vi "ResonanceAnalyzer.vi"() -> ()   [LabVIEW 2014]
uses:
  <vilib>/imath/engines/lvmath2/RunTimeEngine/Managers/WorkSpace/UID Generator.vi
  <vilib>/imathl/engines/lvmath/Functions/Error Handling/Create Error.vi
  <vilib>/imath/engines/lvmath2/RunTimeEngine/LocalVariableDefStatement/MC_LocalVariableDefStatement_Display.vi
  <vilib>/imath/engines/lvmath2/RunTimeEngine/RunTimeType/NIMS_RunTimeType_From StrictType (excl LVString).vi
  <vilib>/imath/engines/lvmath2/RunTimeEngine/BuiltInFunctions/length/NIMS_length(GV).vi
  <vilib>/imath/engines/lvmath2/RunTimeEngine/BuiltInFunctions/ones/NIMS_V=ones(I32,I32).vi
  <vilib>/imath/engines/lvmath2/RunTimeEngine/IndexRead/NIMS V(S).vi
  <vilib>/imath/engines/lvmath2/RunTimeEngine/ErrorHandling/NIMS_Create Error From Enums.vi
  <vilib>/imath/engines/lvmath2/RunTimeEngine/CommandStatement/MC_CommandStatement_break.vi
  <vilib>/imath/engines/lvmath2/RunTimeEngine/Managers/SymbolTable/Clear UID.vi
  <vilib>/imath/engines/lvmath2/RunTimeEngine/Managers/SymbolTable/NIMS_WorkSpace.lvlib
  <vilib>/imath/engines/lvmath2/RunTimeEngine/NodeEndStatement/NIMS_NodeEndStatement_Output.vi
  <vilib>/imath/engines/lvmath2/RunTimeEngine/ErrorHandling/NIMS_Finalize Error.vi
  <vilib>/imath/engines/lvmath2/RunTimeEngine/IndexReplace/NIMS V(S)=S.vi
  <vilib>/Utility/file.llb/Read From Spreadsheet File (DBL).vi
  <vilib>/imath/engines/lvmath2/RunTimeEngine/RangeToken/NIMS_Range_R2 - Integer.vi
  <vilib>/imath/engines/lvmath2/RunTimeEngine/BuiltInFunctions/transpose/NIMS_transpose(GV).vi
  <vilib>/imath/engines/lvmath2/RunTimeEngine/RangeToken/NIMS_Range.vi
  <vilib>/Analysis/NI_AALBase.lvlib
  <vilib>/gmath/NI_Gmath.lvlib
  <vilib>/gmath/NumericalOptimization/Nonlinear Curve Fit LM formula string.vi
panel:
  out "best nonlinear fit":dbl[](array[numeric])
  out "f":dbl[](array[numeric])
  out "A":dbl[](array[numeric])
  out "XY Graph":cluster{"Y":dbl[], "Y":dbl[]}[](graph)
  in  "?":enum32{"Simulation", "Experiment"}(tab)
  in  "Input Parameters":T1
  in  "Filename":path
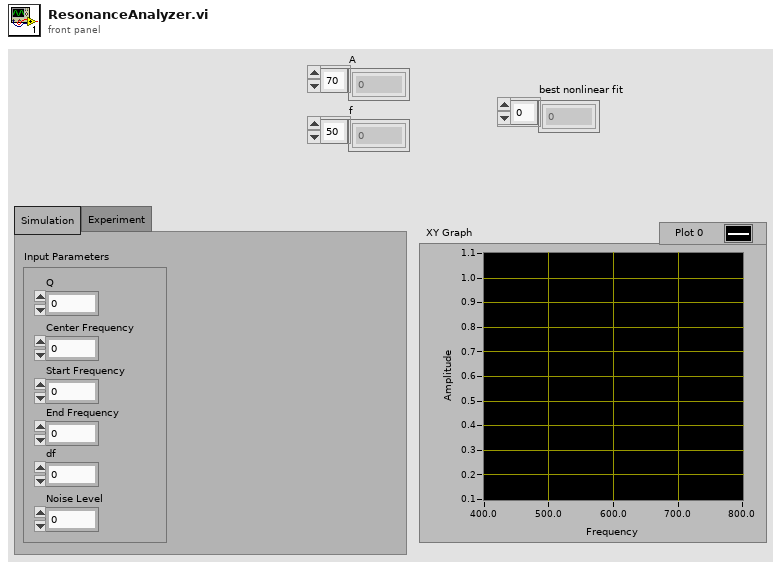
[diagram p1: front panel]
types:
  T1 = cluster{"Q":dbl, "Center Frequency":dbl, "Start Frequency":dbl, "End Frequency":dbl, "df":dbl, "Noise Level":dbl}
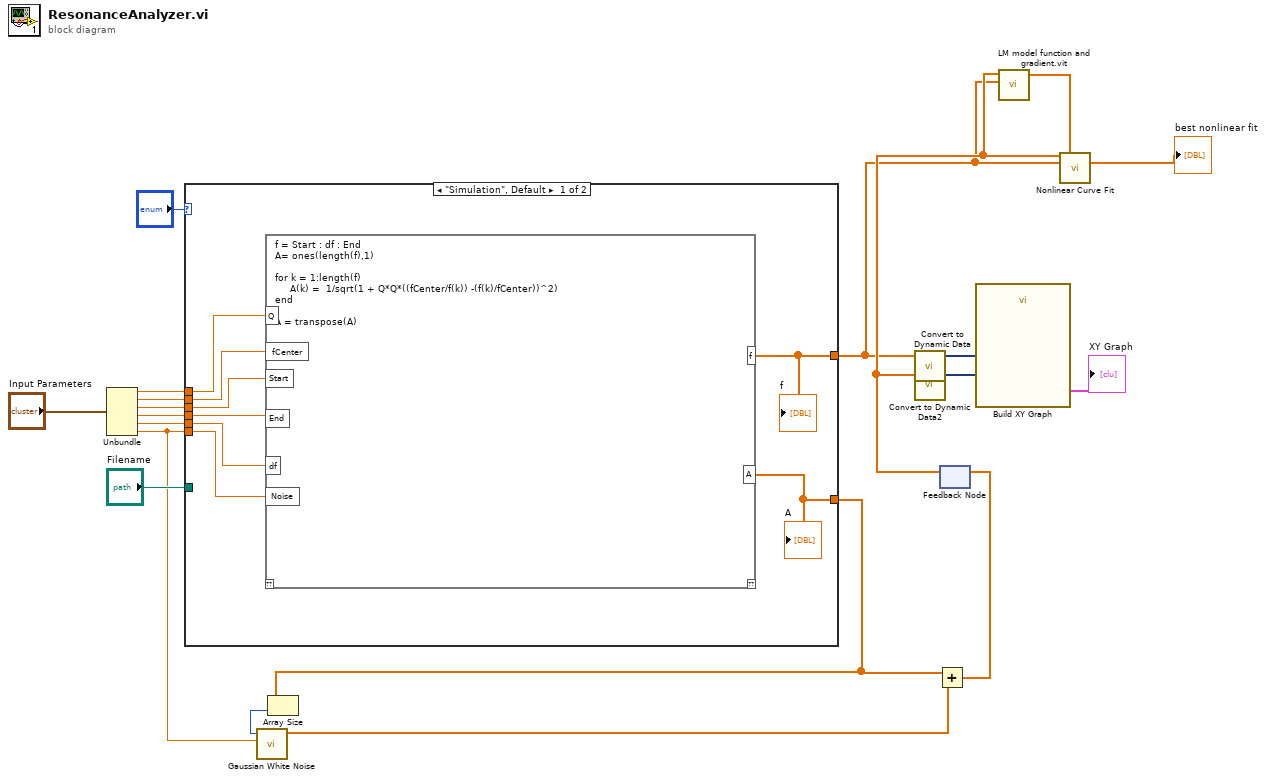
[diagram p0: block diagram]
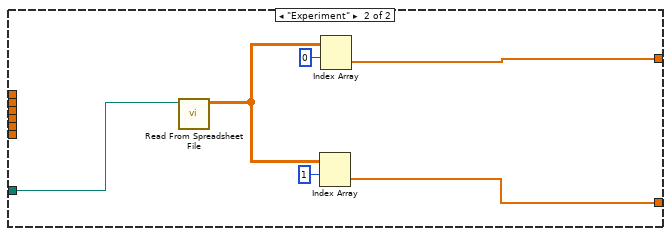
[diagram p2: hidden frame]
diagram:
  n1 = Unbundle("Input Parameters") -> ("Q"=w18:dbl, "Center Frequency"=w17:dbl, "Start Frequency"=w16:dbl, "End Frequency"=w15:dbl, "df"=w14:dbl, "Noise Level"=w9:dbl)
  n2 = case shown="\"Simulation\", Default" "?" {
    tunnel: w18 -> [w28 _]
    tunnel: w17 -> [w27 _]
    tunnel: w16 -> [w26 _]
    tunnel: w15 -> [w25 _]
    tunnel: w14 -> [w24 _]
    tunnel: w9 -> [w23 _]
    tunnel: "Filename" -> [_ w227]
    tunnel: [w21 w223] -> w1
    tunnel: [w22 w222] -> w4
    frame "Simulation", Default {
      n3 = mathscript code="f = Start : df : End\nA= ones(length(f),1)\n\nfor k = 1:length(f)\n     A(k) =  1/sqrt(1 + Q*Q*((fCenter/f(k)) -(f(k)/fCenter))^2)\nend\n\nA = transpose(A)"("fCenter"=w27, "Q"=w28, "Start"=w26, "End"=w25, "df"=w24, "Noise"=w23) -> ("A"=w22:dbl[], "f"=w21:dbl[])  [unwired: 1 in, 1 out]
      "A" <- w22
      "f" <- w21
    }
    frame "Experiment" {
      n4 = call-poly <vilib>:"Read From Spreadsheet File.vi"("file path (dialog if empty)"=w227) -> ("all rows"=w224:dbl[][])  [unwired: 6 in, 4 out]
      n5 = Index Array(array=w224, index (row)=1 ("index")) -> (element=w222:dbl[])  [unwired: 1 in]
      n6 = Index Array(array=w224, index (row)=0 ("index")) -> (element=w223:dbl[])  [unwired: 1 in]
    }
  }
  n7 = Array Size(array=w4) -> (size(s)=w8:i32)
  n8 = call <vilib>:"Gaussian White Noise.vi"("standard deviation"=w9, "samples"=w8) -> ("Gaussian noise pattern"=w7:dbl[])  [unwired: 8 in, 1 out]
  n9 = call "Convert to Dynamic Data"("Array"=w1) -> ("Dynamic Data Type"=w11:dynamicdata)  [unwired: 3 in]
  n10 = Add(x=w4, y=w7) -> (x+y=w6:dbl[])
  n11 = feedback-in #1(w6) -> ()
  n12 = feedback #1() -> (w2:dbl[])  [unwired: 1 in]
  n13 = call "Convert to Dynamic Data2"("Array"=w2) -> ("Dynamic Data Type"=w10:dynamicdata)  [unwired: 3 in]
  n14 = call "Build XY Graph"("Y Input"=w10, "X Input"=w11) -> ("XY Graph"=→"XY Graph":cluster{"X":dbl[], "Y":dbl[]}[])  [unwired: 8 in, 1 out]
  n15 = call <vilib>:"LM model function and gradient.vit"("X"=w1, "a"=w2) -> ("f(X,a)"=w3:dbl[])  [unwired: 2 in, 2 out]
  n16 = call-poly <vilib>:"Nonlinear Curve Fit.vi"("Y"=w2, "initial parameters"=w3, "X"=w1) -> ("best fit parameters"=→"best nonlinear fit":dbl[])  [unwired: 8 in, 4 out]
